vi "read pyro tcp.vi"(8 "error in (no error)":errorcluster, 11 "TCP Network Connection in":refnum<k5>) -> (0 "error out":errorcluster, 2 "readout":dbl[](array[numeric]), 3 "TCP Network Connection out":refnum<k5>)   [LabVIEW 2020, in "TCPClient.lvclass"]
uses:
  TCPClient.lvclass
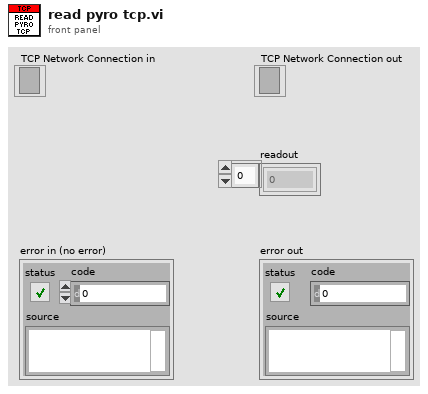
[diagram p1: front panel]
types:
  T1 = enum16{"Standard", "Buffered", "CRLF", "Immediate"}
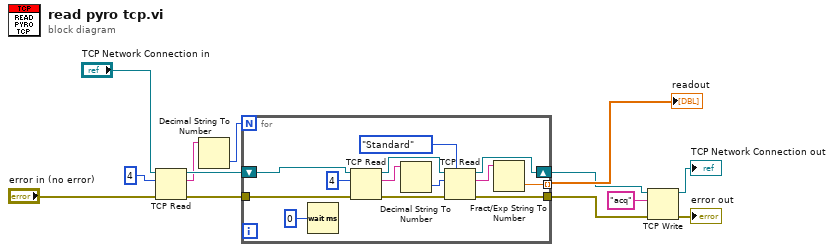
[diagram p0: block diagram]
diagram:
  n1 = TCP Read(connection ID="TCP Network Connection in", bytes to read=4, error in (no error)="error in (no error)") -> (connection ID out=w8:refnum<k5>, data out=w7:string, error out=w12:errorcluster)  [unwired: 2 in]
  n2 = Decimal String To Number(string=w7) -> (number=w6:i32)  [unwired: 2 in, 1 out]
  n3 = for {
    N: w6 -> [_]
    shift-right: [w21] -> w3
    shift-left: w8 -> [w17]
    tunnel: [w18] -> w13 mode=indexing
    tunnel: w12 -> [w16]
    tunnel: [w14] -> w4
    n4 = Wait (ms)(milliseconds to wait=u32 0) -> ()  [unwired: 1 out]
    n5 = TCP Read(connection ID=w17, bytes to read=4, error in (no error)=w16) -> (connection ID out=w24:refnum<k5>, data out=w22:string, error out=w15:errorcluster)  [unwired: 2 in]
    n6 = Decimal String To Number(string=w22) -> (number=w20:i32)  [unwired: 2 in, 1 out]
    n7 = TCP Read(connection ID=w24, bytes to read=w20, error in (no error)=w15, 7:T1."Standard" ("mode (standard)")) -> (connection ID out=w21:refnum<k5>, data out=w19:string, error out=w14:errorcluster)  [unwired: 1 in]
    n8 = Fract/Exp String To Number(string=w19) -> (number=w18:dbl)  [unwired: 3 in, 1 out]
  }
  "readout" <- w13
  n9 = TCP Write(connection ID=w3, data in="acq", error in (no error)=w4) -> (connection ID out=→"TCP Network Connection out":refnum<k5>, error out=→"error out":errorcluster)  [unwired: 1 in, 1 out]
